vi "DEMO-Read STM32F103RB ID.vi"() -> ()   [LabVIEW 2016]
uses:
  <userlib>/LV-JLinkARM/JLinkARM.lvlib
panel:
  out "buff out":string
  in  "停止":bool
  out "error out":errorcluster
  in  "error in (no error)":errorcluster caption="错误输入（无错误）"
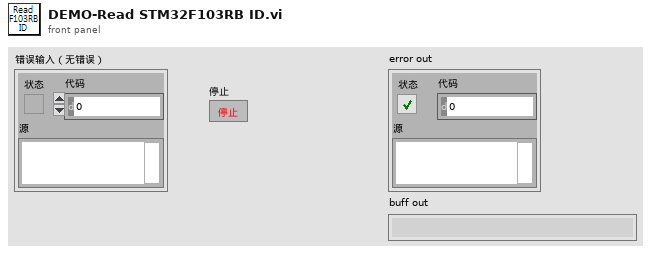
[diagram p1: front panel]
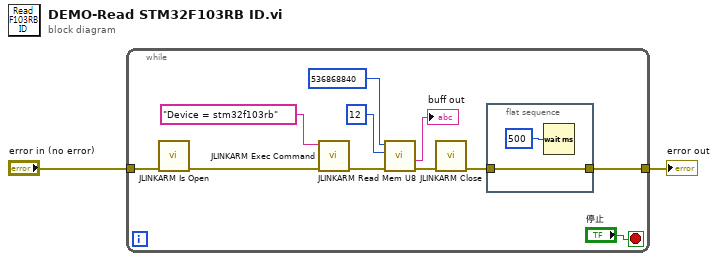
[diagram p0: block diagram]
diagram:
  n1 = while {
    tunnel: "error in (no error)" -> [w10]
    tunnel: [w9] -> w1
    stop <- "停止" stop-if-true
    n2 = call <userlib>:"JLINKARM Is Open.vi"("error in (no error)"=w10) -> ("error out"=w13:errorcluster)  [unwired: 9 in, 1 out]
    n3 = call <userlib>:"JLINKARM Exec Command.vi"("error in (no error)"=w13, "pbCommand"="Device = stm32f103rb") -> ("error out"=w12:errorcluster)  [unwired: 7 in, 2 out]
    n4 = call <userlib>:"JLINKARM Read Mem U8.vi"("error in (no error)"=w12, "size"=u32 12, "memaddr"=u32 536868840) -> ("error out"=w11:errorcluster, "buff out"=→"buff out":string)  [unwired: 6 in, 1 out]
    n5 = call <userlib>:"JLINKARM Close.vi"("error in (no error)"=w11) -> ("error out"=w8:errorcluster)  [unwired: 9 in, 1 out]
    n6 = flat-sequence {
      tunnel: [w14] -> w9
      tunnel: w8 -> [w14]
      frame #0 {
        n7 = Wait (ms)(milliseconds to wait=u32 500 ("等待时间（毫秒）")) -> ()  [unwired: 1 out]
      }
    }
  }
  "error out" <- w1
